vi "Create FP Item.vi"(6 "Cluster Component":bool, 8 "error in (no error)":errorcluster, 10 "GObject In":refnum<vi>, 11 "GObject in":refnum<class "Object.lvclass">) -> (0 "error out":errorcluster, 1 "Is Control":bool, 2 "Is Indicator":bool, 3 "GObject out":refnum<class "Object.lvclass">, 4 "All Objects Created":refnum<class "Object.lvclass">[](array[class]), 5 "Is Visible":bool)   [LabVIEW 2017, in "Front Panel Publisher.lvlib" / "Object.lvclass"]
uses:
  Object.lvclass
  Attributes.ctl
  Coordinates.ctl
  <vilib>/Utility/miscctls.llb/LVRectTypeDef.ctl
  Enum - Pane Coordinate Method.ctl
  Front Panel Publisher.lvlib
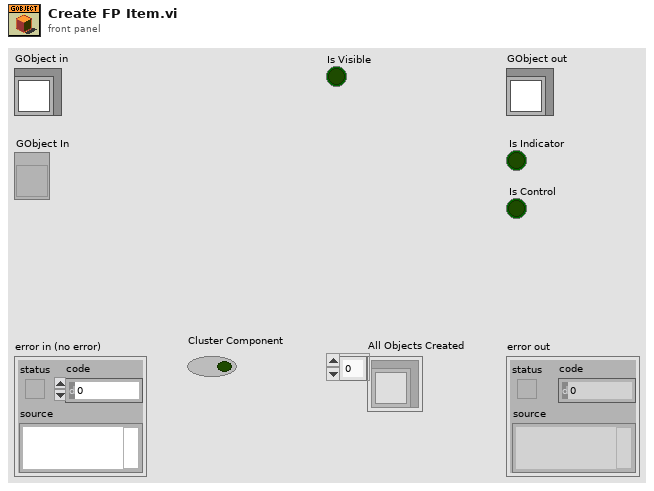
[diagram p1: front panel]
types:
  T1 = typedef "Front Panel Publisher.lvlib/Object.lvclass/Enum - Pane Coordinate Method.ctl" = enum16{"Initialize", "Get Last Pane Offset", "Update Pane Position"}
  T2 = typedef "Front Panel Publisher.lvlib/Object.lvclass/Attributes.ctl" = cluster{"UID":i32, "Type":string, "Starting Location":T3, "Reference":refnum<vi>, "Cluster Component":bool, "Starting Rect Position":cluster{"Left":i16, "Top":i16}, "Owning Pane":refnum<vi>, "Master Total Rect Delta":T4}
  T3 = typedef "Front Panel Publisher.lvlib/Object.lvclass/Coordinates.ctl" = cluster{"Left":i32, "Top":i32, "Height":u32, "Width":u32}
  T4 = typedef "LVRectTypeDef.ctl" = cluster{"Left":i16, "Top":i16, "Right":i16, "Bottom":i16}
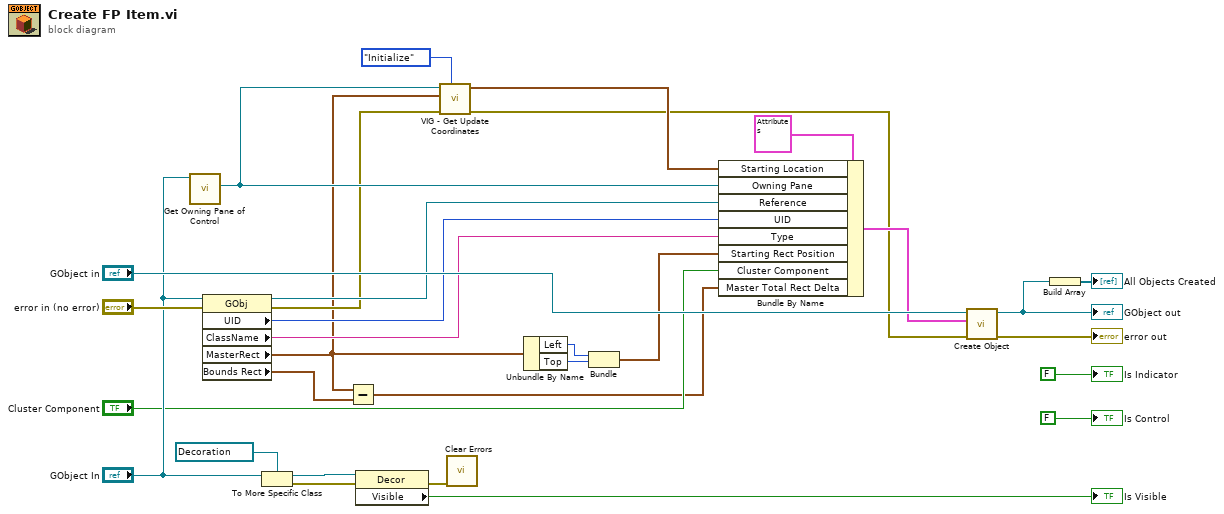
[diagram p0: block diagram]
diagram:
  n1 = call "Get Owning Pane of Control.vi"("GObj Refnum"="GObject In") -> ("Owning Pane"=w7:refnum<vi>)  [unwired: 7 in, 3 out]
  n2 = property class="GObj"(reference="GObject In", error in="error in (no error)") -> (reference out=w13:refnum<vi>, error out=w6:errorcluster, "UID"=w15:i32, "ClassName"=w14:string, "MasterRect"=w4:T4, "Bounds Rect"=w3:T4)
  n3 = To More Specific Class(target class=refnum<vi> refnum ("GOject"), reference="GObject In") -> (specific class reference=w29:refnum<vi>, error out=w28:errorcluster)  [unwired: 1 in]
  n4 = Subtract(x=w4, y=w3) -> (x-y=w2:T4)
  n5 = property class="Decor"(reference=w29, error in=w28) -> (error out=w27:errorcluster, "Visible"=→"Is Visible":bool)  [unwired: 1 out]
  n6 = call "VIG - Get Update Coordinates.vi"("Pane Method"=Enum_-_Pane_Coordinate_Method."Initialize", "error in (no error)"=w6, "MasterRect"=w4, "Pane in"=w7) -> ("error out"=w5:errorcluster, "Coordinates"=w8:T3)  [unwired: 5 in, 1 out]
  n7 = call <vilib>:"Clear Errors.vi"("error in (no error)"=w27) -> ()  [unwired: 5 in, 2 out]
  n8 = Unbundle By Name(w4) -> ("Left"=w11:i16, "Top"=w10:i16)
  n9 = Bundle("Left"=w11, "Top"=w10) -> (w9:cluster{"Left":i16, "Top":i16})  [unwired: 1 in]
  n10 = Bundle By Name(cluster=T2 {"UID"=0, "Type"="", "Starting Location"={"Left"=0, "Top"=0, "Height"=0, "Width"=0}, "Reference"=refnum, "Cluster Component"=FALSE, "Starting Rect Position"={"Left"=0, "Top"=0}, "Owning Pane"=refnum, "Master Total Rect Delta"={"Left"=0, "Top"=0, "Right"=0, "Bottom"=0}} ("Object Attributes"), "Starting Location"=w8, "Owning Pane"=w7, "Reference"=w13, "UID"=w15, "Type"=w14, "Starting Rect Position"=w9, "Cluster Component"="Cluster Component", "Master Total Rect Delta"=w2) -> (w16:T2)
  n11 = call-dynamic "Create Object.vi"("error in (no error)"=w5, "Object Attributes"=w16, "GObject in"="GObject in") -> ("error out"=→"error out":errorcluster, "GObject out"=w20:refnum<class "Object.lvclass">)  [unwired: 7 in]
  "GObject out" <- w20
  n12 = Build Array(w20) -> (→"All Objects Created":refnum<class "Object.lvclass">[])
  "Is Indicator" <- FALSE ("Is Indicator")
  "Is Control" <- FALSE ("Is Control")
